vi "Test Noise Buffer Length.vi"(8 "error in (no error)":errorcluster, 11 "SR7270 Drivers in":refnum<class "SR7270 Drivers.lvclass">) -> (0 "error out":errorcluster, 3 "SR7270 Drivers out":refnum<class "SR7270 Drivers.lvclass">)   [LabVIEW 2016, in "SR7270 Drivers.lvclass"]
uses:
  SR7270 Drivers.lvclass
  Typedefs/NNBUF--enum.ctl
  <vilib>/addons/_JKI Toolkits/Caraya/classes/Assert/Assert.lvclass
  <vilib>/addons/_JKI Toolkits/Caraya/classes/Test/Test.lvclass
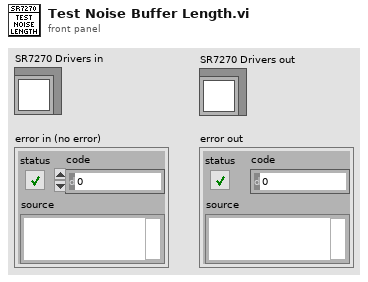
[diagram p1: front panel]
types:
  T1 = typedef "SR7270 Drivers.lvclass/NNBUF--enum.ctl" = enum16{"Off", "1 seconds", "2 seconds", "3 seconds", "4 seconds"}
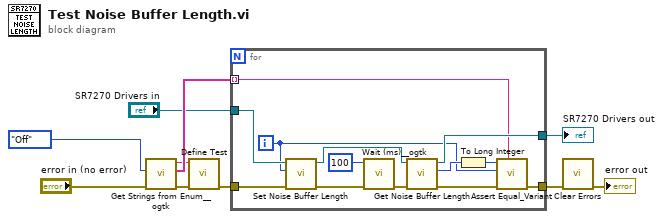
[diagram p0: block diagram]
diagram:
  n1 = call <userlib>:"Get Strings from Enum__ogtk.vi"("error in (no error)"="error in (no error)", "Enum"=NNBUF--enum."Off" ("Noise Buffer Length")) -> ("error out"=w4:errorcluster, "Enum Strings"=w7:string[], "Enum Name"=w5:string)  [unwired: 6 in, 1 out]
  n2 = call <vilib>:"Define Test.vi"("error in (no error)"=w4, "Label (VI Title)"=w5) -> ("error out"=w2:errorcluster)  [unwired: 9 in]
  n3 = for {
    tunnel: "SR7270 Drivers in" -> [w22]
    tunnel: w2 -> [w14]
    tunnel: [w20] -> w10
    tunnel: [w19] -> w9
    tunnel: w7 -> [w11] mode=indexing
    i -> [w13]
    n4 = call "Set Noise Buffer Length.vi"("error in (no error)"=w14, "Noise Buffer Length"=w13, "SR7270 Drivers in"=w22) -> ("error out"=w16:errorcluster, "SR7270 Drivers out"=w23:refnum<class "SR7270 Drivers.lvclass">)  [unwired: 7 in]
    n5 = call <userlib>:"Wait (ms)__ogtk.vi"("error in (no error)"=w16, "milliseconds to wait"=u32 100) -> ("error out"=w18:errorcluster)  [unwired: 8 in, 1 out]
    n6 = call "Get Noise Buffer Length.vi"("error in (no error)"=w18, "SR7270 Drivers in"=w23) -> ("error out"=w21:errorcluster, "Noise Buffer Length"=w15:T1, "SR7270 Drivers out"=w19:refnum<class "SR7270 Drivers.lvclass">)  [unwired: 7 in]
    n7 = To Long Integer(number=w15) -> (32bit integer=w12:i32)
    n8 = call <vilib>:"Assert Equal_Variant.vi"("Label"=w11, "error in (no error)"=w21, "Y"=w13, "X"=w12) -> ("error out"=w20:errorcluster)  [unwired: 7 in]
  }
  "SR7270 Drivers out" <- w9
  n9 = call <vilib>:"Clear Errors.vi"("error in (no error)"=w10) -> ("error out"=→"error out":errorcluster)  [unwired: 5 in, 1 out]
